vi "Read PowerSV.vi"(8 "error in (no error)":errorcluster, 11 "FlipMir in":refnum<class "FlipMir.lvclass">) -> (0 "error out":errorcluster, 2 "PowerSV":refnum<k21>, 3 "FlipMir out":refnum<class "FlipMir.lvclass">)   [LabVIEW 2016, in "FlipMir.lvclass"]
uses:
  FlipMir.lvclass
  FlipMir.lvclass/FlipMir.ctl
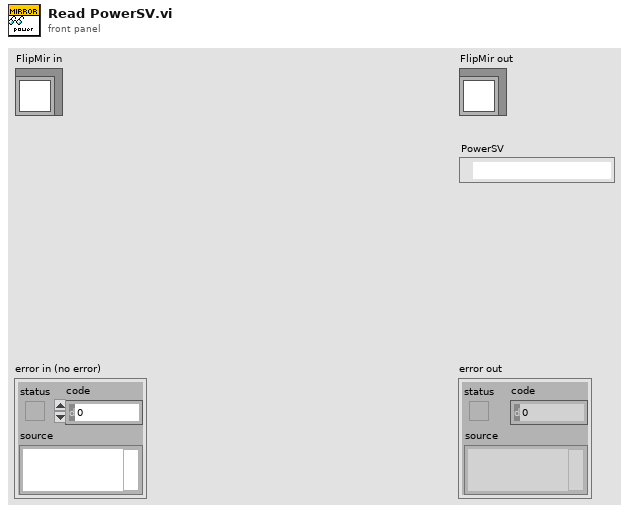
[diagram p1: front panel]
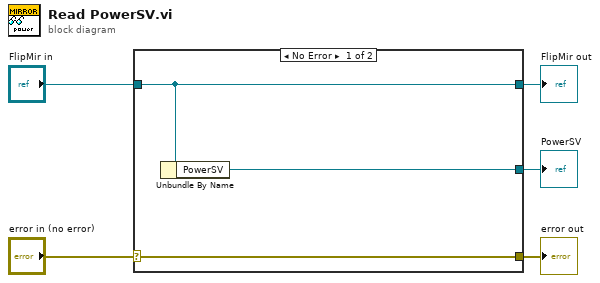
[diagram p0: block diagram]
diagram:
  n1 = case shown="No Error" "error in (no error)" {
    selector: "error in (no error)" -> [w8 w9]
    tunnel: [w8 w9] -> w4
    tunnel: [w7 w10] -> w2
    tunnel: "FlipMir in" -> [w7 w10]
    tunnel: [w6 _] -> w1
    frame No Error {
      n2 = Unbundle By Name(w7) -> ("PowerSV"=w6:refnum<k21>)
    }
    frame Error {
    }
  }
  "error out" <- w4
  "FlipMir out" <- w2
  "PowerSV" <- w1
